vi "LWXPS_PositionerCorrectorNotchFiltersGet.vi"(0 "XPS Reference IN":refnum<k24>, 2 "Positioner Name":string, 5 "LabVIEW error IN":errorcluster) -> (10 "XPS Reference OUT":refnum<k24>, 11 "LabVIEW error OUT":errorcluster, 12 "Returned error code":i32, 13 "XPS Error String":string, 14 "Notch Frequency 1":dbl, 15 "Notch Bandwidth 1":dbl, 16 "Notch Gain 1":dbl, 17 "Notch Frequency 2":dbl, 18 "Notch Bandwidth 2":dbl, 19 "Notch Gain 2":dbl)   [LabVIEW 2014]
uses:
  D:/XPSQ8_LabView_Library/Development/Source/Dll/Newport.XPS.CommandInterface.dll
  Dll/Newport.XPS.CommandInterface.dll
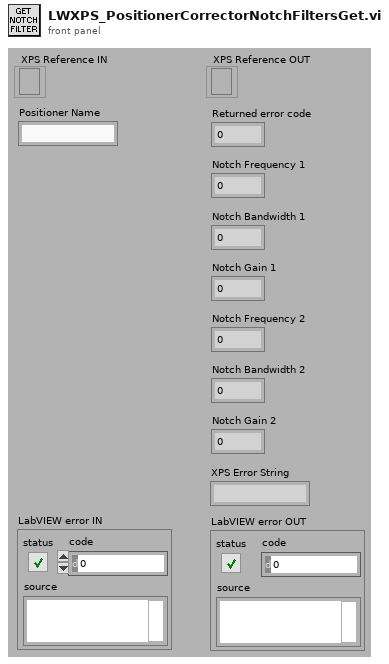
[diagram p1: front panel]
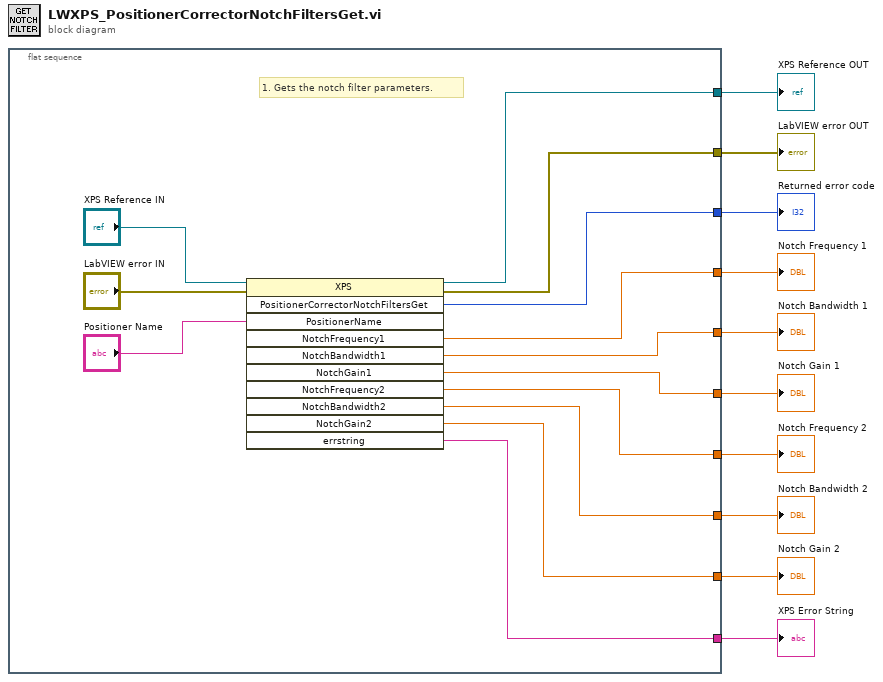
[diagram p0: block diagram]
diagram:
  n1 = flat-sequence {
    tunnel: [w21] -> w10
    tunnel: [w18] -> w9
    tunnel: [w22] -> w8
    tunnel: [w13] -> w1
    tunnel: [w16] -> w7
    tunnel: [w17] -> w4
    tunnel: [w15] -> w6
    tunnel: [w14] -> w5
    tunnel: [w12] -> w3
    tunnel: [w11] -> w2
    frame #0 {
      # "1. Gets the notch filter parameters."
      n2 = invoke class="XPS" method="PositionerCorrectorNotchFiltersGet"(reference="XPS Reference IN", error in="LabVIEW error IN", "PositionerName"="Positioner Name") -> (reference out=w21:refnum<k24>, error out=w18:errorcluster, "PositionerCorrectorNotchFiltersGet"=w22:i32, "NotchFrequency1"=w13:dbl, "NotchBandwidth1"=w16:dbl, "NotchGain1"=w15:dbl, "NotchFrequency2"=w14:dbl, "NotchBandwidth2"=w17:dbl, "NotchGain2"=w12:dbl, "errstring"=w11:string)  [unwired: 8 in, 1 out]
    }
  }
  "XPS Error String" <- w2
  "XPS Reference OUT" <- w10
  "LabVIEW error OUT" <- w9
  "Returned error code" <- w8
  "Notch Bandwidth 1" <- w7
  "Notch Gain 1" <- w6
  "Notch Frequency 2" <- w5
  "Notch Bandwidth 2" <- w4
  "Notch Gain 2" <- w3
  "Notch Frequency 1" <- w1
